vi "GET_ALL_ISSUES.vi"() -> ()   [LabVIEW 2024]
uses:
  <vilib>/addons/_JKI.lib/Serialization/JSON/JKI JSON Serialization.lvlib
  <vilib>/addons/_JKI.lib/REST Client/classes/REST Client/REST Client.lvclass
panel:
  out "days left":dbl
  out "Hours left":dbl
  out "status":bool
  out "retries":i32=4
  in  "jail time (min)":dbl=10.0 caption="Delay Time (s)"
  in  "Delay Time (s)":dbl=18.0
  out "progress":i32(slide)=4825 caption="3526 of 29182" scale=0.0..29182.0
  in  "error in (no error)":errorcluster
  out "error out":errorcluster
  in  "issues path":path=path "D:/Comics/data/cv_issues"
  out "current file":string=" (1903) #"
  in  "volumes path":path=path "D:/Comics/data/cv_volumes"
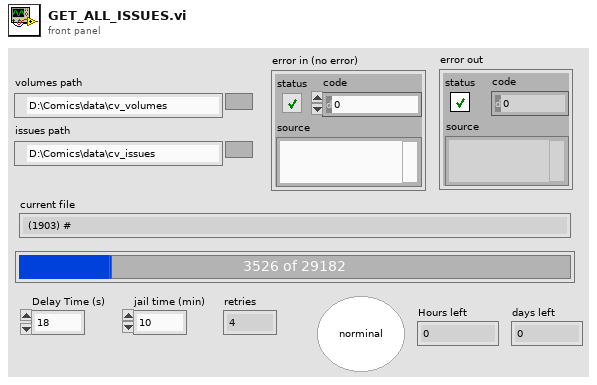
[diagram p1: front panel]
types:
  T1 = enum16{"open", "replace", "create", "open or create", "replace or create", "replace or create with confirmation"}
  T2 = typedef "local_issue.ctl" = cluster{"cover_date":timestamp, "id":i32, "cv_id":string, "name":string, "sortable_name":string, "issue_number":string, "deck":string, "description":string, "volume":T3, "store_date":timestamp, "date_last_updated":timestamp, "site_detail_url":string, "cover_url":string, "associated_images":T4[], "characters":T3[], "concepts":T3[], "creators":T5[], "storyArcs":T3[], "teams":T3[]}
  T3 = typedef "comicvine_issue.generic_credit.ctl" = cluster{"id":i32, "name":string}
  T4 = typedef "comicvine_issue.associated_image.ctl" = cluster{"original_url":string, "id":i32}
  T5 = typedef "comicvine_issue.person_credit.ctl" = cluster{"id":i32, "name":string, "role":string}
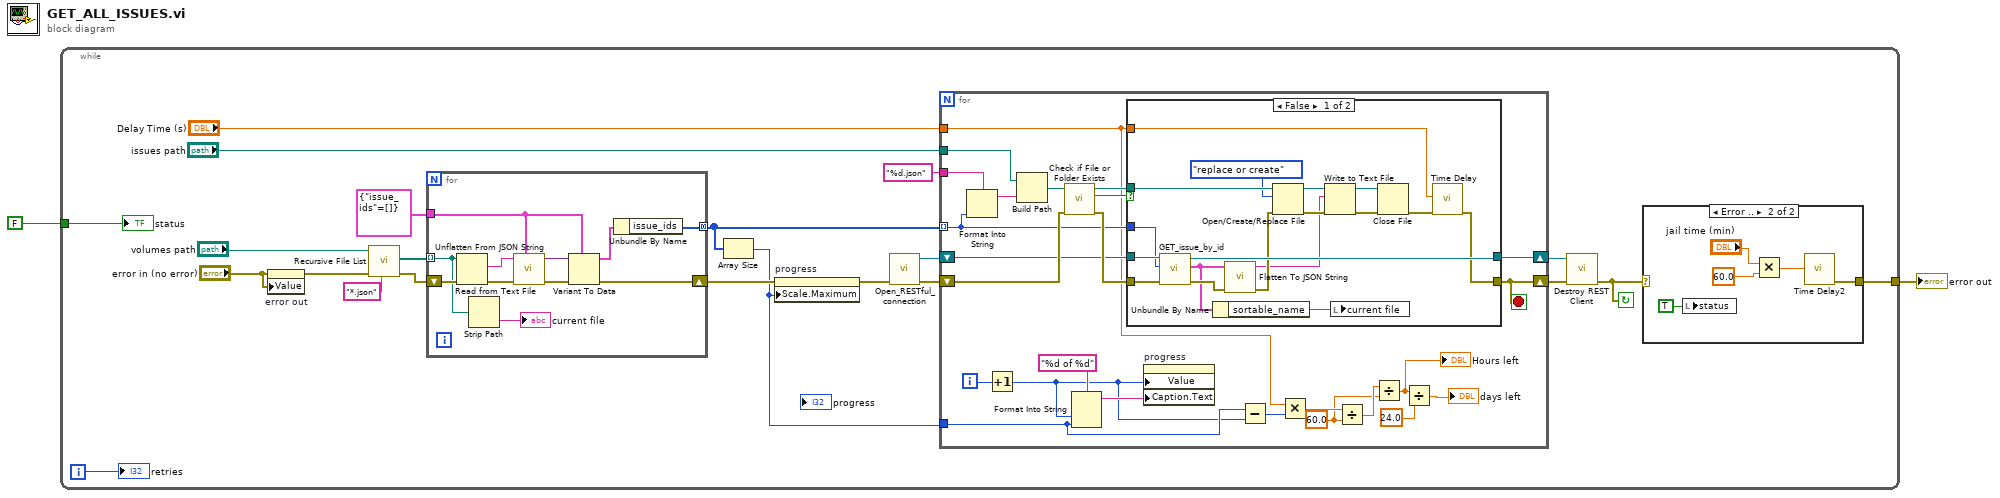
[diagram p0: block diagram]
diagram:
  n1 = while {
    tunnel: [w8] -> w2
    tunnel: FALSE -> [w6]
    i -> [w7]
    stop <- w3 continue-if-true
    n2 = property on="error out" class="Clust (strict)"(error in="error in (no error)", "Value"="error in (no error)") -> (error out=w14:errorcluster)  [unwired: 1 in, 1 out]
    n3 = call <vilib>:"Recursive File List.vi"("pattern"="*.json", "error in (no error)"=w14, "Folder Path"="volumes path") -> ("error out"=w21:errorcluster, "All Files in Dir"=w23:path[])  [unwired: 4 in, 3 out]
    n4 = for {
      tunnel: w23 -> [w77] mode=indexing
      shift-right: [w81] -> w12
      shift-left: w21 -> [w86]
      tunnel: cluster{"issue_ids":i32[]} {"issue_ids"=[]} -> [w82]
      tunnel: [w79] -> w13 mode=concatenating
      n5 = Read from Text File(file (use dialog)=w77, error in=w86) -> (text=w78:string, error out=w85:errorcluster)  [unwired: 2 in, 2 out]
      n6 = Strip Path(path=w77) -> (name=→"current file":string)  [unwired: 1 out]
      n7 = call <vilib>:"Unflatten From JSON String.vi"("Type and Defaults"=w82, "error in"=w85, "JSON String"=w78) -> ("error out"=w84:errorcluster, "Variant"=w83:variant)  [unwired: 7 in]
      n8 = Variant To Data(error in=w84, type=w82, Variant=w83) -> (data=w80:cluster{"issue_ids":i32[]}, error out=w81:errorcluster)
      n9 = Unbundle By Name(w80) -> ("issue_ids"=w79:i32[])
    }
    n10 = Array Size(array=w13) -> (size(s)=w10:i32)
    n11 = property on="progress" class="Slide (strict)"(error in=w12, "Scale.Maximum"=w10) -> (error out=w11:errorcluster)  [unwired: 1 in, 1 out]
    n12 = call "Open_RESTful_connection.vi"("error in (no error)"=w11) -> ("error out"=w19:errorcluster, "REST Client out"=w18:refnum<class "REST Client.lvclass">)  [unwired: 9 in]
    n13 = for {
      tunnel: w13 -> [w45] mode=indexing
      shift-right: [w41] -> w4
      shift-left: w19 -> [w51]
      shift-right: [w47] -> w5
      shift-left: w18 -> [w46]
      tunnel: "issues path" -> [w54]
      tunnel: "%d.json" ("format string") -> [w53]
      tunnel: w10 -> [w40]
      tunnel: "Delay Time (s)" -> [w37]
      i -> [w44]
      stop <- w41 stop-if-true
      w34 = 60.0 ("y")
      n14 = Format Into String(format string=w53, w45) -> (resulting string=w55:string)  [unwired: 2 in, 1 out]
      n15 = Increment(x=w44) -> (x+1=w39:i32)
      n16 = Build Path(base path=w54, name or relative path=w55) -> (appended path=w52:path)
      n17 = call <vilib>:"Check if File or Folder Exists.vi"("error in (no error)"=w51, "path"=w52) -> ("error out"=w49:errorcluster, "file or folder exists?"=w50:bool, "dup path"=w48:path)  [unwired: 7 in]
      n18 = Format Into String(format string="%d of %d", w39, w40) -> (resulting string=w42:string)  [unwired: 2 in, 1 out]
      n19 = case shown="False" w50 {
        tunnel: [w59 w75] -> w41
        tunnel: w49 -> [w72 w75]
        tunnel: w48 -> [w68 _]
        tunnel: [w70 w74] -> w47
        tunnel: w46 -> [w73 w74]
        tunnel: w45 -> [w71 _]
        tunnel: w37 -> [w56 _]
        frame False {
          n20 = call "GET_issue_by_id.vi"("error in (no error)"=w72, "issue id"=w71, "REST Client in"=w73) -> ("error out"=w69:errorcluster, "local_issue"=w58:T2, "REST Client out"=w70:refnum<class "REST Client.lvclass">)  [unwired: 6 in]
          n21 = Unbundle By Name(w58) -> ("sortable_name"=w57:string)
          n22 = call <vilib>:"Flatten To JSON String.vi"("error in"=w69, "Variant"=w58) -> ("error out"=w67:errorcluster, "JSON String"=w64:string)  [unwired: 8 in]
          n23 = Open/Create/Replace File(file path (use dialog)=w68, error in=w67, operation (0:open)=T1."replace or create") -> (refnum out=w63:refnum<file>, error out=w65:errorcluster)  [unwired: 3 in, 1 out]
          n24 = Write to Text File(file (use dialog)=w63, text=w64, error in=w65) -> (refnum out=w61:refnum<file>, error out=w62:errorcluster)  [unwired: 1 in, 1 out]
          n25 = local write "current file"(w57) -> ()
          n26 = Close File(refnum=w61, error in=w62) -> (error out=w60:errorcluster)  [unwired: 1 out]
          n27 = call "Time Delay"("error in (no error)"=w60, "Delay Time (s)"=w56) -> ("error out"=w59:errorcluster)  [unwired: 9 in]
        }
        frame True {
        }
      }
      n28 = property on="progress" class="Slide (strict)"("Value"=w39, "Caption.Text"=w42) -> ()  [unwired: 2 in, 2 out]
      n29 = Subtract(x=w40, y=w39) -> (x-y=w38:i32)
      n30 = Multiply(x=w37, y=w38) -> (x*y=w36:dbl)
      n31 = Divide(x=w36, y=w34) -> (x/y=w35:dbl)
      n32 = Divide(x=w35, y=w34) -> (x/y=w33:dbl)
      "Hours left" <- w33
      n33 = Divide(x=w33, y=24.0) -> (x/y=→"days left":dbl)
    }
    n34 = call-dynamic "Destroy REST Client.vi"("error in (no error)"=w4, "REST Client in"=w5) -> ("error out"=w3:errorcluster)  [unwired: 9 in]
    n35 = case shown="Error .." w3 {
      selector: w3 -> [w25 _]
      tunnel: [w25 w30] -> w8
      frame No Error {
      }
      frame Error {
        n36 = local write "status"(TRUE ("status")) -> ()
        n37 = Multiply(x="jail time (min)", y=60.0) -> (x*y=w27:dbl)
        n38 = call "Time Delay2"("Delay Time (s)"=w27) -> ("error out"=w30:errorcluster)  [unwired: 10 in]
      }
    }
    "retries" <- w7
    "status" <- w6
  }
  "error out" <- w2
